vi "nav run.vi"(9 "Drone":T2, 10 "nav type":i32, 11 "Field":T3[][](array[typedef])) -> (2 "Move?":bool, 3 "direction":T1 items=["^", "^>", ">", "V>", "V", "<V", "<", "<^"])   [LabVIEW 2009]
uses:
  square.ctl
  Drone data.ctl
  direction.ctl
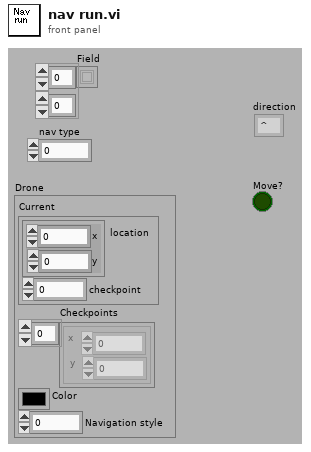
[diagram p1: front panel]
types:
  T1 = typedef "direction.ctl" = i8
  T2 = typedef "Drone data.ctl" = cluster{"Current":cluster{"location":cluster{"x":i16, "y":i16}, "checkpoint":i32}, "Checkpoints":cluster{"x":i16, "y":i16}[], "Color":u32, "Navigation style":i32}
  T3 = typedef "square.ctl" = u8
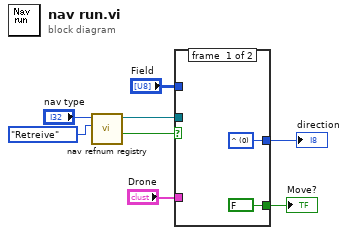
[diagram p0: block diagram]
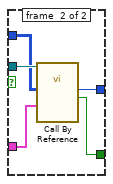
[diagram p2: hidden frame]
diagram:
  n1 = call "nav refnum registry.vi"("Action"=enum16{"Open", "Retreive", "Close"}."Retreive", "nav type"="nav type") -> ("valid refnum?"=w1:bool, "VI reference"=w6:refnum<vi>)  [unwired: 8 in]
  n2 = case shown="True" w1 {
    tunnel: w6 -> [_ w15]
    tunnel: "Field" -> [_ w14]
    tunnel: "Drone" -> [_ w13]
    tunnel: [w9 w12] -> w3
    tunnel: [FALSE ("Move?") w11] -> w2
    frame #0 {
      w9 = T1 0 items=["^", "^>", ">", "V>", "V", "<V", "<", "<^"] ("direction")
    }
    frame #1 {
      n3 = call-by-ref "?"(reference=w15, "Drone"=w13, "Field"=w14) -> ("Move?"=w11:bool, "direction"=w12:T1)  [unwired: 9 in, 2 out]
    }
  }
  "direction" <- w3
  "Move?" <- w2
